vi "buildTestLog.vi"(8 "error in (no error)":errorcluster, 9 "Serial Number":string, 10 "TestLogTypes":T1, 11 "ITestLogFactory in":refnum<class "ITestLogFactory.lvclass">) -> (0 "error out":errorcluster, 2 "ITestLog":refnum<class "ITestLog.lvclass">, 3 "ITestLogFactory out":refnum<class "ITestLogFactory.lvclass">)   [LabVIEW 2015, in "ITestLogFactory.lvclass"]
uses:
  ITestLogFactory.lvclass
  Typedefs/TestLogTypes.ctl
  TestLog/ITestLog/ITestLog.lvclass
  Typedefs/FAMTTypedefs.lvlib
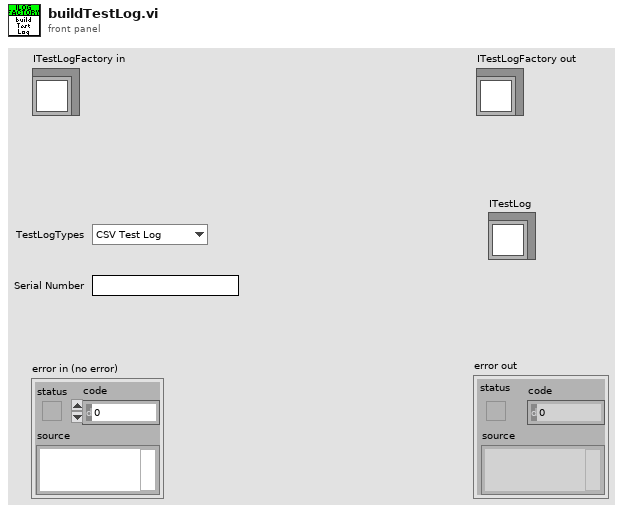
[diagram p1: front panel]
types:
  T1 = typedef "FAMTTypedefs.lvlib/TestLogTypes.ctl" = enum16{"CSV Test Log"}
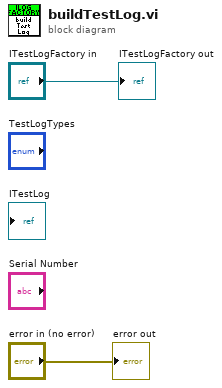
[diagram p0: block diagram]
diagram:
  "error out" <- "error in (no error)"
  "ITestLogFactory out" <- "ITestLogFactory in"
